vi "Encoders.vi"(3 "Reset All":bool) -> (0 "Avg Absolute Rate":dbl, 1 "Avg Absolute Distance":dbl)   [LabVIEW 2014]
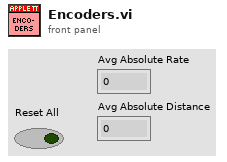
[diagram p1: front panel]
types:
  T1 = typedef "WPI_EncoderDevRef.ctl" = cluster{"DevStatus":errorcluster, "EncoderIndex":T2, "CounterIndex":T3, "DistancePerCount":dbl, "Decoding Type":T4}
  T2 = typedef "FPGA_EncoderIdx.ctl" = enum8{"Enc 0", "Enc 1", "Enc 2", "Enc 3", "Enc 4", "Enc 5", "Enc 6", "Enc 7", "Invalid"}
  T3 = typedef "FPGA_CounterCtrSystemIndex.ctl" = enum8{"Ctr 0", "Ctr 1", "Ctr 2", "Ctr 3", "Ctr 4", "Ctr 5", "Ctr 6", "Ctr 7", "Invalid"}
  T4 = typedef "WPI_EncoderType.ctl" = enum16{"1x", "2x", "4x"}
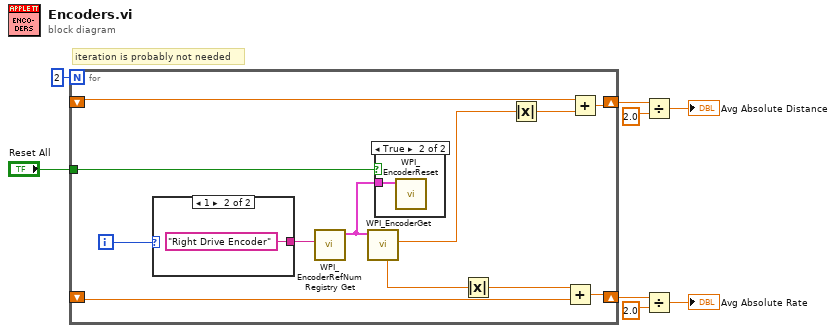
[diagram p0: block diagram]
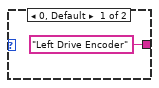
[diagram p3: hidden frame]
diagram:
  # "iteration is probably not needed"
  n1 = for {
    N: 2 -> [_]
    shift-right: [w19] -> w2
    shift-left: _ -> [w18]
    tunnel: "Reset All" -> [w16]
    shift-right: [w13] -> w6
    shift-left: _ -> [w12]
    i -> [w9]
    n2 = case shown="1" w9 {
      tunnel: ["Left Drive Encoder" ("refnum name") "Right Drive Encoder" ("refnum name")] -> w20
      frame 0, Default {
      }
      frame 1 {
      }
    }
    n3 = call <vilib>:"WPI_EncoderRefNum Registry Get.vi"("refnum name"=w20) -> ("EncoderDevRef"=w17:T1)  [unwired: 9 in, 1 out]
    n4 = call <vilib>:"WPI_EncoderGet.vi"("EncoderDevRef"=w17) -> ("Distance"=w10:dbl, "Rate"=w11:dbl)  [unwired: 5 in, 4 out]
    n5 = case shown="True" w16 {
      tunnel: w17 -> [_ w21]
      frame False {
      }
      frame True {
        n6 = call <vilib>:"WPI_EncoderReset.vi"("EncoderDevRef"=w21) -> ()  [unwired: 9 in, 2 out]
      }
    }
    n7 = Absolute Value(x=w11) -> (abs(x)=w15:dbl)
    n8 = Absolute Value(x=w10) -> (abs(x)=w14:dbl)
    n9 = Add(x=w15, y=w18) -> (x+y=w19:dbl)
    n10 = Add(x=w12, y=w14) -> (x+y=w13:dbl)
  }
  n11 = Divide(x=w6, y=2.0) -> (x/y=→"Avg Absolute Distance":dbl)
  n12 = Divide(x=w2, y=2.0) -> (x/y=→"Avg Absolute Rate":dbl)
